vi "Generate MAX Report.vi"(6 "Overwrite (F)":bool, 8 "error in (no error)":errorcluster, 9 "Report Type (XML)":T1 items=["XML", "HTML", "Technical Support"], 10 "Output Filename":path, 11 "Session in":refnum<k21>="localhost") -> (0 "error out":errorcluster, 3 "Session out":refnum<k21>)   [LabVIEW 2020, in "nisyscfg.lvlib"]
doc: "Creates a report to document a local or remote system. Reports can be generated in three formats: XML, HTML, and technical support reports.\n\nBoth HTML and XML formats provide readable reports. The XML format makes archiving and comparing reports convenient with a configuration management tool. The technical support format generates a ZIP file containing reports that are useful if you need to contact NI Technical Support. The level of support for this VI depends on each device's driver software. This function provides a one-way export only. You cannot import the XML-based report into MAX."
uses:
  <vilib>/nisyscfg/nisyscfg.lvlib
  <vilib>/nisyscfg/Report Mode.ctl
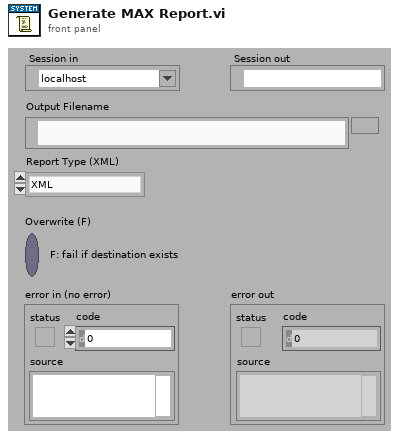
[diagram p1: front panel]
types:
  T1 = typedef "nisyscfg.lvlib/Report Mode.ctl" = i32
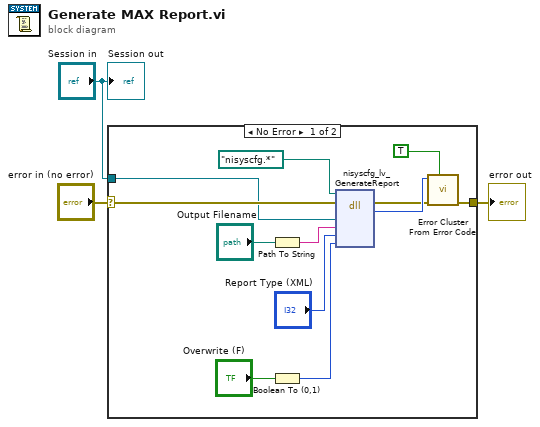
[diagram p0: block diagram]
diagram:
  n1 = case shown="No Error" "error in (no error)" {
    selector: "error in (no error)" -> [w7 w16]
    tunnel: [w14 w16] -> w3
    tunnel: "Session in" -> [w6 _]
    frame No Error {
      n2 = Path To String(path="Output Filename") -> (string=w10:string)
      n3 = Boolean To (0,1)(Boolean="Overwrite (F)") -> (0, 1=w8:i16)
      n4 = dll-call lib="nisyscfg.*" fn="nisyscfg_lv_GenerateReport" label="GenerateReport"(path in=path "nisyscfg.*", error in=w7, "sessionHandle"=w6, "outputFilename"=w10, "reportType"="Report Type (XML)", "overwriteIfExists"=w8) -> (error out=w11:errorcluster, "return type"=w12:i32)  [unwired: 5 in, 1 out]
      n5 = call <vilib>:"Error Cluster From Error Code.vi"("show call chain? (False)"=TRUE, "error in (no error)"=w11, "error code (0)"=w12) -> ("error out"=w14:errorcluster)  [unwired: 6 out]
    }
    frame Error {
    }
  }
  "error out" <- w3
  "Session out" <- "Session in"
